vi "Intialize.vi"(7 "On Chip Accumulations 3":i32=6, 8 "error in (no error)":errorcluster, 9 "Time between frames 2":i32=500, 10 "Number of Frames 3":i32, 11 "VISA resource name":refnum<visa-resource-name>="COM7") -> (0 "error out":errorcluster, 3 "VISA resource name out":refnum<visa-resource-name>)   [LabVIEW 2018]
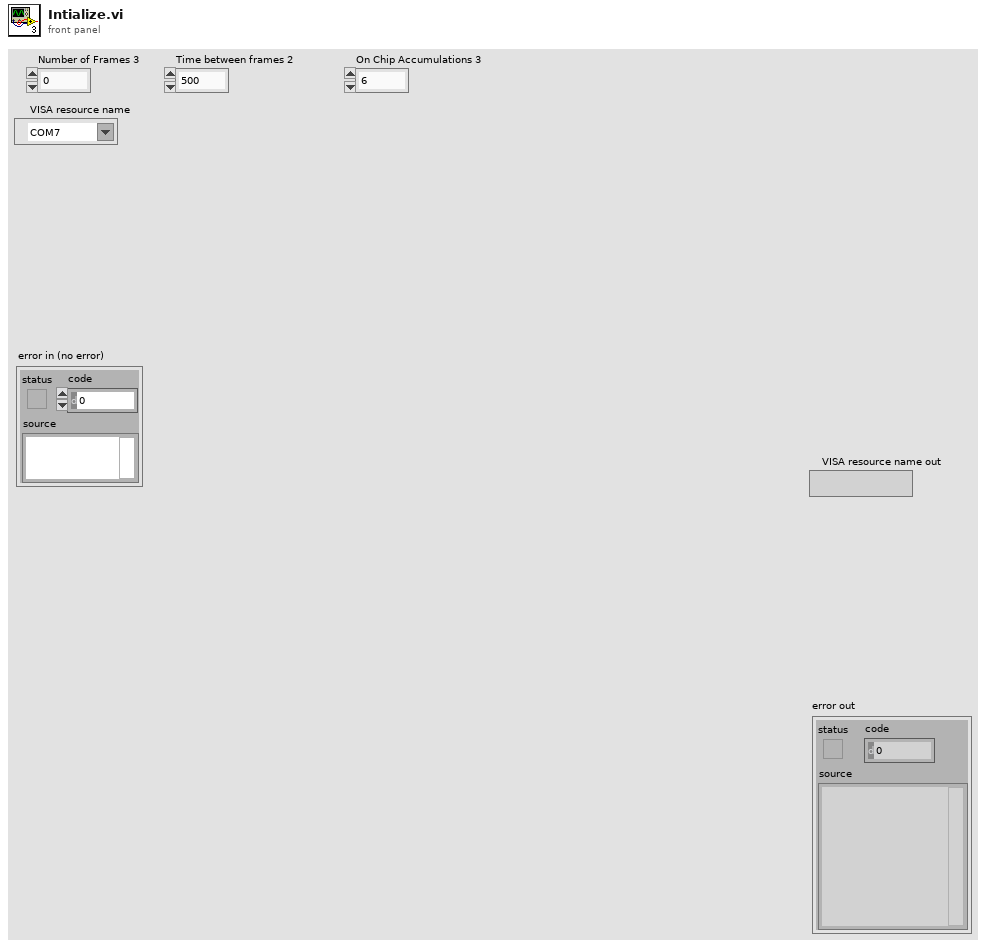
[diagram p1: front panel]
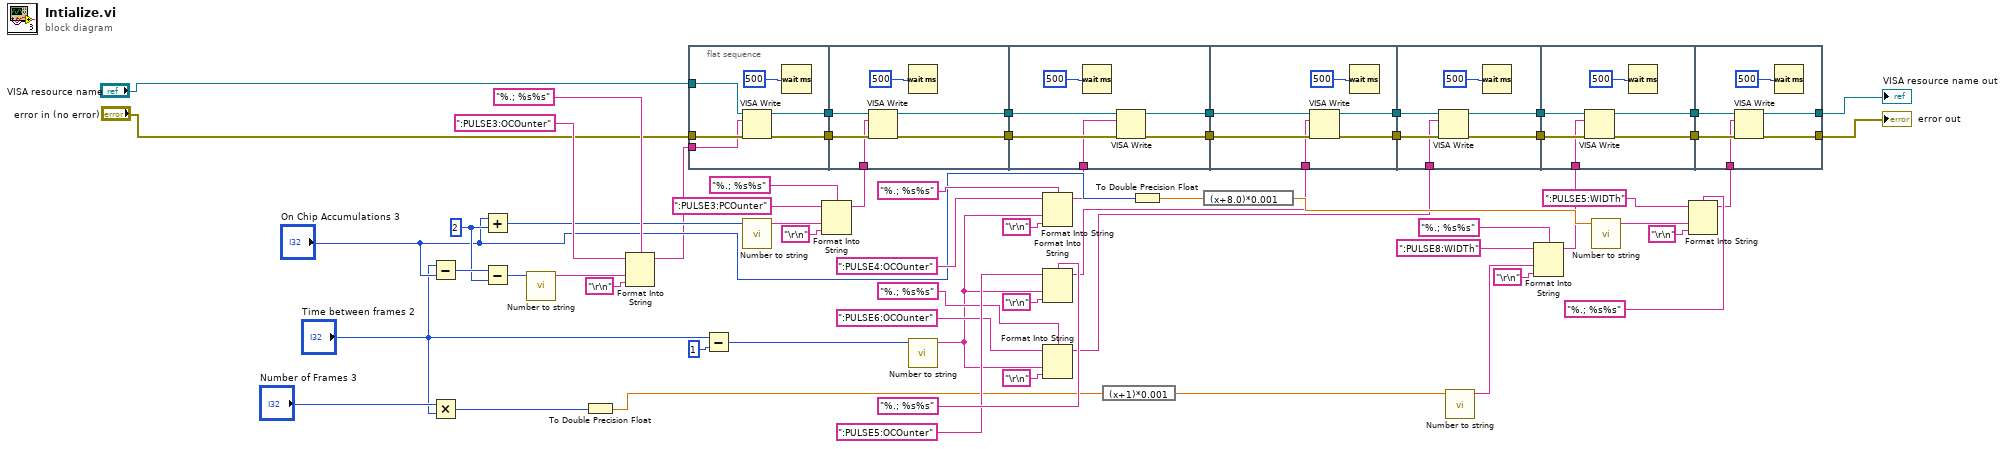
[diagram p0: block diagram]
diagram:
  w45 = 2 ("y")
  n1 = Subtract(x="Time between frames 2", y="On Chip Accumulations 3") -> (x-y=w47:i32)
  n2 = Multiply(x="Number of Frames 3", y="Time between frames 2") -> (x*y=w12:i32)
  n3 = Add(x="On Chip Accumulations 3", y=w45) -> (x+y=w41:i32)
  n4 = Subtract(x=w47, y=w45) -> (x-y=w46:i32)
  n5 = call "Number to string.vi"("Numeric"=w46) -> ("Shortest String"=w51:string)  [unwired: 10 in]
  n6 = To Double Precision Float(number=w12) -> (double precision float=w27:dbl)
  n7 = Format Into String(format string="%.; %s%s", initial string=":PULSE3:OCOunter" ("format string"), w51, "\r\n" ("format string")) -> (resulting string=w11:string)  [unwired: 1 in, 1 out]
  n8 = flat-sequence {
    tunnel: "error in (no error)" -> [w69]
    tunnel: w11 -> [w68]
    tunnel: "VISA resource name" -> [w67]
    tunnel: [w66] -> w63
    tunnel: [w65] -> w62
    tunnel: w63 -> [w74]
    tunnel: w10 -> [w73]
    tunnel: w62 -> [w72]
    tunnel: [w71] -> w61
    tunnel: [w70] -> w60
    tunnel: w61 -> [w81]
    tunnel: w9 -> [w80]
    tunnel: w60 -> [w79]
    tunnel: [w78] -> w59
    tunnel: [w77] -> w58
    tunnel: w59 -> [w87]
    tunnel: w8 -> [w86]
    tunnel: w58 -> [w85]
    tunnel: [w84] -> w57
    tunnel: [w83] -> w56
    tunnel: w57 -> [w93]
    tunnel: w7 -> [w92]
    tunnel: w56 -> [w91]
    tunnel: [w90] -> w55
    tunnel: [w89] -> w54
    tunnel: w55 -> [w99]
    tunnel: w6 -> [w98]
    tunnel: w54 -> [w97]
    tunnel: [w96] -> w53
    tunnel: [w95] -> w52
    tunnel: w53 -> [w105]
    tunnel: w5 -> [w104]
    tunnel: w52 -> [w103]
    tunnel: [w101] -> w2
    tunnel: [w100] -> w1
    frame #0 {
      n9 = VISA Write(VISA resource name=w67, write buffer=w68, error in (no error)=w69) -> (VISA resource name out=w65:refnum<visa-resource-name>, error out=w66:errorcluster)  [unwired: 1 out]
      n10 = Wait (ms)(milliseconds to wait=500) -> ()  [unwired: 1 out]
    }
    frame #1 {
      n11 = VISA Write(VISA resource name=w72, write buffer=w73, error in (no error)=w74) -> (VISA resource name out=w70:refnum<visa-resource-name>, error out=w71:errorcluster)  [unwired: 1 out]
      n12 = Wait (ms)(milliseconds to wait=500) -> ()  [unwired: 1 out]
    }
    frame #2 {
      n13 = Wait (ms)(milliseconds to wait=500) -> ()  [unwired: 1 out]
      n14 = VISA Write(VISA resource name=w79, write buffer=w80, error in (no error)=w81) -> (VISA resource name out=w77:refnum<visa-resource-name>, error out=w78:errorcluster)  [unwired: 1 out]
    }
    frame #3 {
      n15 = VISA Write(VISA resource name=w85, write buffer=w86, error in (no error)=w87) -> (VISA resource name out=w83:refnum<visa-resource-name>, error out=w84:errorcluster)  [unwired: 1 out]
      n16 = Wait (ms)(milliseconds to wait=500) -> ()  [unwired: 1 out]
    }
    frame #4 {
      n17 = VISA Write(VISA resource name=w91, write buffer=w92, error in (no error)=w93) -> (VISA resource name out=w89:refnum<visa-resource-name>, error out=w90:errorcluster)  [unwired: 1 out]
      n18 = Wait (ms)(milliseconds to wait=500) -> ()  [unwired: 1 out]
    }
    frame #5 {
      n19 = VISA Write(VISA resource name=w97, write buffer=w98, error in (no error)=w99) -> (VISA resource name out=w95:refnum<visa-resource-name>, error out=w96:errorcluster)  [unwired: 1 out]
      n20 = Wait (ms)(milliseconds to wait=500) -> ()  [unwired: 1 out]
    }
    frame #6 {
      n21 = VISA Write(VISA resource name=w103, write buffer=w104, error in (no error)=w105) -> (VISA resource name out=w101:refnum<visa-resource-name>, error out=w100:errorcluster)  [unwired: 1 out]
      n22 = Wait (ms)(milliseconds to wait=500) -> ()  [unwired: 1 out]
    }
  }
  n23 = Subtract(x="Time between frames 2", y=1) -> (x-y=w38:i32)
  n24 = call "Number to string.vi"("Numeric"=w41) -> ("Shortest String"=w44:string)  [unwired: 10 in]
  n25 = Format Into String(format string="%.; %s%s", initial string=":PULSE3:PCOunter" ("format string"), w44, "\r\n" ("format string")) -> (resulting string=w10:string)  [unwired: 1 in, 1 out]
  n26 = call "Number to string.vi"("Numeric"=w38) -> ("Shortest String"=w28:string)  [unwired: 10 in]
  n27 = Format Into String(format string="%.; %s%s", initial string=":PULSE4:OCOunter" ("format string"), w28, "\r\n" ("format string")) -> (resulting string=w9:string)  [unwired: 1 in, 1 out]
  n28 = Format Into String(format string="%.; %s%s", initial string=":PULSE5:OCOunter" ("format string"), w28, "\r\n" ("format string")) -> (resulting string=w8:string)  [unwired: 1 in, 1 out]
  n29 = Format Into String(format string="%.; %s%s", initial string=":PULSE6:OCOunter" ("format string"), w28, "\r\n" ("format string")) -> (resulting string=w7:string)  [unwired: 1 in, 1 out]
  n30 = expression code="(x+1)*0.001"(w27) -> (w24:dbl)
  n31 = To Double Precision Float(number="On Chip Accumulations 3") -> (double precision float=w20:dbl)
  n32 = expression code="(x+8.0)*0.001"(w20) -> (w15:dbl)
  n33 = call "Number to string.vi"("Numeric"=w24) -> ("Shortest String"=w23:string)  [unwired: 10 in]
  n34 = Format Into String(format string="%.; %s%s", initial string=":PULSE8:WIDTh" ("format string"), w23, "\r\n" ("format string")) -> (resulting string=w6:string)  [unwired: 1 in, 1 out]
  n35 = call "Number to string.vi"("Numeric"=w15) -> ("Shortest String"=w17:string)  [unwired: 10 in]
  n36 = Format Into String(format string="%.; %s%s", initial string=":PULSE5:WIDTh" ("format string"), w17, "\r\n" ("format string")) -> (resulting string=w5:string)  [unwired: 1 in, 1 out]
  "error out" <- w1
  "VISA resource name out" <- w2
